vi "DUAL GAUGE-Offset Correction.vi"(7 "W/R":bool, 8 "Fehler (Eingang)":errorcluster, 9 "Sensor 2 Set":u8(ring) items=["off", "on", "auto"], 10 "Sensor 1 Set":u8(ring) items=["off", "on", "auto"], 11 "Referenz in":refnum<visa-resource-name>) -> (0 "Cluster (Ausgang)":errorcluster, 1 "Sensor 2 Get":u8(ring) items=["off", "on", "auto"], 2 "Sensor 1 Get":u8(ring) items=["off", "on", "auto"], 3 "Referenz out":refnum<visa-resource-name>)   [LabVIEW 2013, in "Dual Gauge.lvlib"]
uses:
  Dual Gauge.lvlib
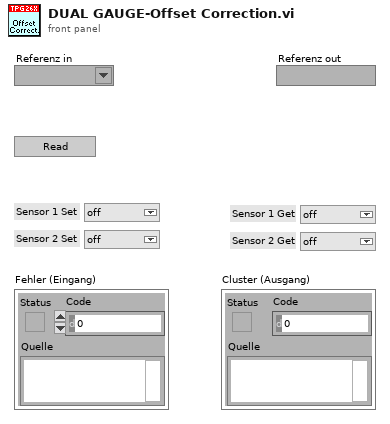
[diagram p1: front panel]
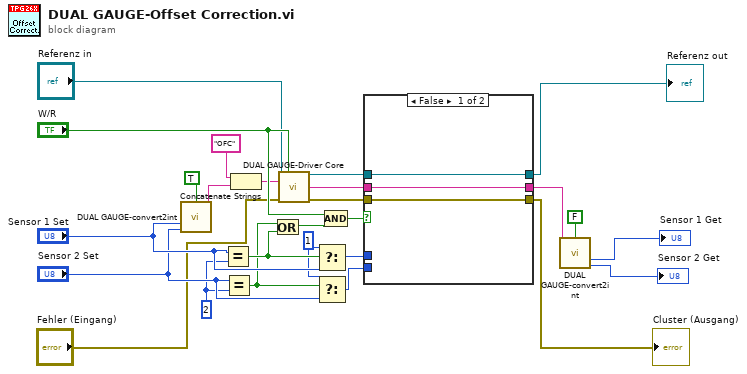
[diagram p0: block diagram]
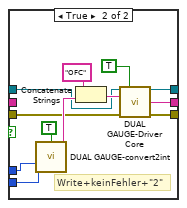
[diagram p2: hidden frame]
diagram:
  w12 = u8 1 ("y")
  w17 = u8 2 ("y")
  n1 = call "DUAL GAUGE-convert2int.vi"("W/R [W: Int in; Str out ]"=TRUE, "Integer1 in"="Sensor 1 Set", "Integer2 in"="Sensor 2 Set") -> ("String out"=w19:string)  [unwired: 8 in, 4 out]
  n2 = Equal?(x="Sensor 1 Set", y=w17) -> (x = y?=w16:bool)
  n3 = Equal?(x="Sensor 2 Set", y=w17) -> (x = y?=w15:bool)
  n4 = Concatenate Strings("OFC", w19) -> (w5:string)
  n5 = Or(x=w15, y=w16) -> (x .or. y?=w14:bool)
  n6 = call "DUAL GAUGE-Driver Core.vi"("Referenz in"="Referenz in", "Write/Read"="W/R", "Command"=w5, "Fehler (Eingang)"="Fehler (Eingang)") -> ("Referenz out"=w6:refnum<visa-resource-name>, "String Out"=w8:string, "Cluster (Ausgang)"=w7:errorcluster)  [unwired: 9 in]
  n7 = Select(t=w12, s=w16, f="Sensor 1 Set") -> (s? t:f=w11:u8)
  n8 = Select(t=w12, s=w15, f="Sensor 2 Set") -> (s? t:f=w10:u8)
  n9 = Compound Arithmetic op=AND("W/R", w14) -> (w13:bool)
  n10 = case shown="False" w13 {
    tunnel: w11 -> [_ w38]
    tunnel: w10 -> [_ w37]
    tunnel: [w29 w36] -> w9
    tunnel: [w28 w35] -> w1
    tunnel: w8 -> [w29 _]
    tunnel: w7 -> [w28 w32]
    tunnel: w6 -> [w27 w31]
    tunnel: [w27 w30] -> w3
    frame False {
    }
    frame True {
      # "Write+keinFehler+\"2\""
      n11 = call "DUAL GAUGE-convert2int.vi"("W/R [W: Int in; Str out ]"=TRUE, "Integer1 in"=w38, "Integer2 in"=w37) -> ("String out"=w40:string)  [unwired: 8 in, 4 out]
      n12 = Concatenate Strings("OFC", w40) -> (w33:string)
      n13 = call "DUAL GAUGE-Driver Core.vi"("Referenz in"=w31, "Write/Read"=TRUE, "Command"=w33, "Fehler (Eingang)"=w32) -> ("Referenz out"=w30:refnum<visa-resource-name>, "String Out"=w36:string, "Cluster (Ausgang)"=w35:errorcluster)  [unwired: 9 in]
    }
  }
  "Referenz out" <- w3
  "Cluster (Ausgang)" <- w1
  n14 = call "DUAL GAUGE-convert2int.vi"("String in"=w9, "W/R [W: Int in; Str out ]"=FALSE) -> ("Integer3 out"=→"Sensor 1 Get":u8, "Integer4 out"=→"Sensor 2 Get":u8)  [unwired: 9 in, 3 out]
